vi "configuration methods.vi"() -> (0 "error out":errorcluster, 2 "modules equal":bool, 3 "channels equal":bool)   [LabVIEW 2013, in "shared memory module tests.lvlib"]
uses:
  shared memory module tests.lvlib
  module/configuration/shared memory module configuration.lvclass
panel:
  out "created channels":i32
  out "configuration channels":i32
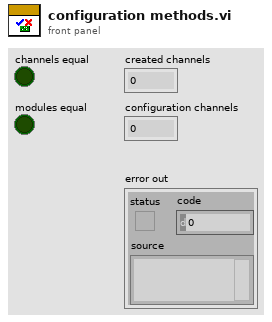
[diagram p1: front panel]
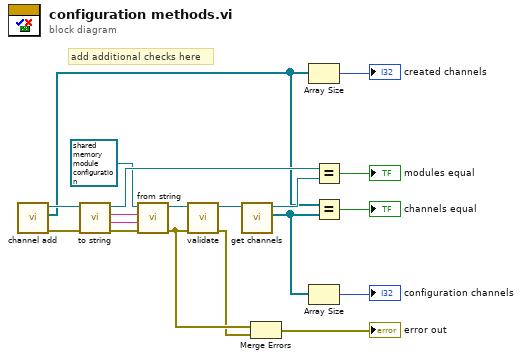
[diagram p0: block diagram]
diagram:
  # "add additional checks here"
  n1 = call "channel add.vi"() -> ("error out"=w12:errorcluster, "channels"=w7:refnum<class "TBM channel.lvclass">[], "configuration out"=w13:refnum<class "shared memory module configuration.lvclass">)  [unwired: 7 in, 2 out]
  n2 = call-dynamic "to string.vi"("error in"=w12, "configuration in"=w13) -> ("error out"=w19:errorcluster, "data"=w18:string, "version"=w17:string, "configuration out"=w9:refnum<class "shared memory module configuration.lvclass">)  [unwired: 6 in]
  n3 = call-dynamic "from string.vi"("error in"=w19, "data"=w18, "version"=w17, "current tag file io module configuration in"=refnum<class "shared memory module configuration.lvclass"> refnum ("tag bus configurable plugin module configuration")) -> ("error out"=w3:errorcluster, "current tag file io module configuration out"=w16:refnum<class "shared memory module configuration.lvclass">)  [unwired: 6 in]
  n4 = call-dynamic "validate.vi"("error in"=w3, "current tag file io module configuration in"=w16) -> ("error out"=w2:errorcluster, "current tag file io module configuration out"=w14:refnum<class "shared memory module configuration.lvclass">)  [unwired: 8 in]
  n5 = call-dynamic "get channels.vi"("current tag file io module configuration in"=w14) -> ("channels"=w6:refnum<class "TBM channel.lvclass">[], "current tag file io module configuration out"=w10:refnum<class "shared memory module configuration.lvclass">)  [unwired: 9 in]
  n6 = Merge Errors(w3, w2) -> (→"error out":errorcluster)
  n7 = Array Size(array=w7) -> (size(s)=→"created channels":i32)
  n8 = Array Size(array=w6) -> (size(s)=→"configuration channels":i32)
  n9 = Equal?(x=w9, y=w10) -> (x = y?=→"modules equal":bool)
  n10 = Equal?(x=w7, y=w6) -> (x = y?=→"channels equal":bool)
